vi "niFpgaInterruptTemplateWithErrorOutput.vi"(1 "Wait Until Cleared":bool, 2 "IRQ Number":u8) -> (0 "Error":bool)   [LabVIEW 2017]
doc: "Asserts an interrupt on the interrupt line of the FPGA target. Support of interrupts and the number of interrupts available varies according to the FPGA target. Refer to the specific FPGA target hardware documentation for more information."
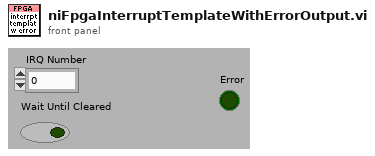
[diagram p1: front panel]
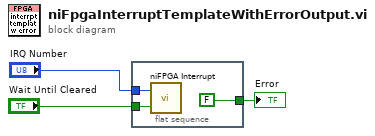
[diagram p0: block diagram]
diagram:
  n1 = flat-sequence {
    tunnel: [FALSE] -> w3
    tunnel: "IRQ Number" -> [w5]
    tunnel: "Wait Until Cleared" -> [w4]
    frame #0 {
      n2 = call <vilib>:"niFPGA Interrupt.vi"("Wait Until Cleared (F)"=w4, "IRQ Number (0)"=w5) -> ()  [unwired: 1 in]
    }
  }
  "Error" <- w3
